vi "Status Update.vi"(8 "error in (no error)":errorcluster, 11 "Stage Controller in":refnum<class "Stage Controller.lvclass">) -> (0 "error out":errorcluster, 3 "Stage Controller out":refnum<class "Stage Controller.lvclass">)   [LabVIEW 2023, in "Stage Controller.lvlib" / "Stage Controller.lvclass"]
uses:
  Stage Controller.lvclass
  Stage Controller.lvclass/Stage Controller.ctl
  <vilib>/ActorFramework/Actor/Actor.lvclass
  Application Messages/Stage Status Msg/Stage Status Msg.lvclass
  Resources/GLOBAL/GLOBAL Experiment Metadata.vi
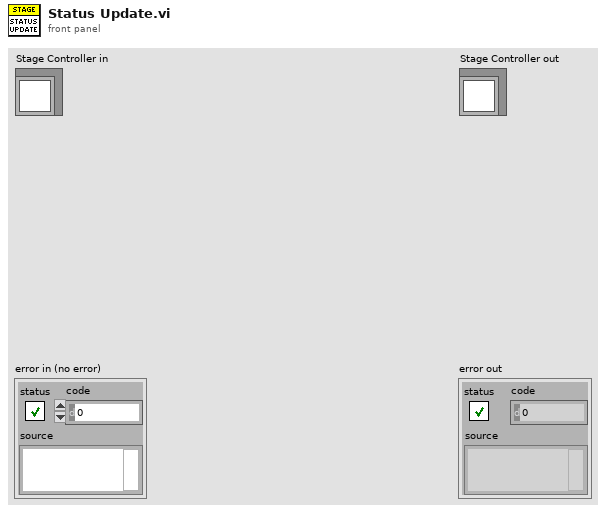
[diagram p1: front panel]
types:
  T1 = cluster{"X (mm)":dbl, "Y (mm)":dbl, "Stage Map":picture}
  T2 = cluster{"Y Min":dbl, "Y Max":dbl, "X Min":dbl, "X Max":dbl}
  T3 = cluster{"top":dbl, "right":dbl, "width":dbl, "height":dbl}
  T4 = typedef "Stage Position.ctl" = cluster{"X (mm)":dbl, "Y (mm)":dbl, "Z (mm)":dbl}
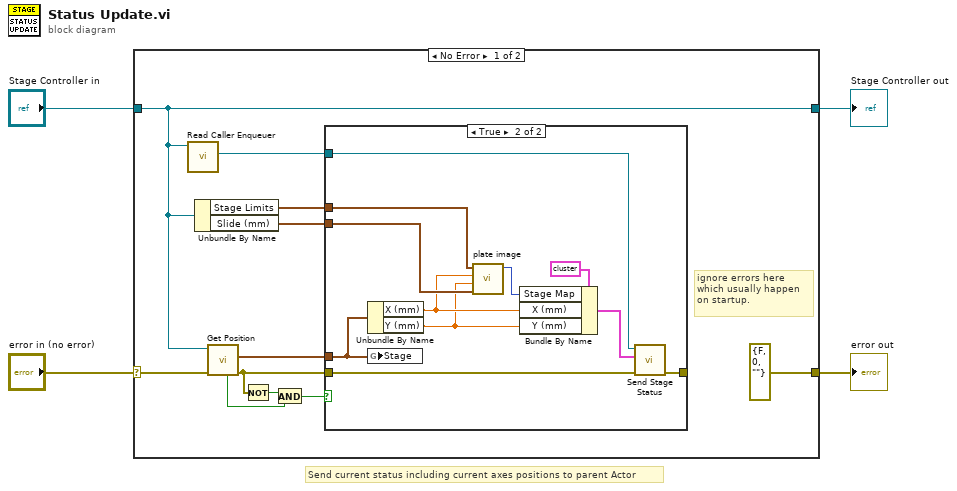
[diagram p0: block diagram]
diagram:
  # "Send current status including current axes positions to parent Actor"
  n1 = case shown="No Error" "error in (no error)" {
    selector: "error in (no error)" -> [w15 w29]
    tunnel: [errorcluster {"status"=FALSE, "code"=0, "source"=""} ("error IO") w29] -> w3
    tunnel: [w9 w28] -> w1
    tunnel: "Stage Controller in" -> [w9 w28]
    frame No Error {
      # "ignore errors here\nwhich usually happen\non startup."
      n2 = call <vilib>:"Read Caller Enqueuer.vi"("Actor"=w9) -> ("Caller Enqueuer"=w14:refnum<class "Message Enqueuer.lvclass">)  [unwired: 10 in]
      n3 = Unbundle By Name(w9) -> ("Stage Limits"=w8:T2, "Slide (mm)"=w5:T3)
      n4 = call-dynamic "Get Position.vi"("error in (no error)"=w15, "Stage Controller in"=w9) -> ("error out"=w13:errorcluster, "Stage Position"=w10:T4, "Value Changed?"=w11:bool)  [unwired: 6 in, 1 out]
      n5 = Not(x=w13) -> (.not. x?=w12:bool)
      n6 = And(x=w12, y=w11) -> (x .and. y?=w7:bool)
      n7 = case shown="True" w7 {
        tunnel: w14 -> [_ w27]
        tunnel: [w16 w25] -> _
        tunnel: w13 -> [w16 w24]
        tunnel: w10 -> [_ w19]
        tunnel: w8 -> [_ w21]
        tunnel: w5 -> [_ w20]
        frame False {
        }
        frame True {
          n8 = Unbundle By Name(w19) -> ("X (mm)"=w18:dbl, "Y (mm)"=w17:dbl)
          n9 = global write "GLOBAL Experiment Metadata.vi" "Stage"(w19) -> ()
          n10 = call "plate image.vi"("Slide (mm)"=w20, "Y (um)"=w17, "X (um)"=w18, "Stage Limits (mm)"=w21) -> ("2D Picture"=w22:picture)  [unwired: 7 in]
          n11 = Bundle By Name(cluster=T1 {"X (mm)"=0.0, "Y (mm)"=0.0, "Stage Map"=bytes[0]} ("Stage Status"), "Stage Map"=w22, "X (mm)"=w18, "Y (mm)"=w17) -> (w26:T1)
          n12 = call "Send Stage Status.vi"("error in (no error)"=w24, "Stage Status"=w26, "Message Enqueuer"=w27) -> ("error out"=w25:errorcluster)  [unwired: 7 in, 1 out]
        }
      }
    }
    frame Error {
    }
  }
  "error out" <- w3
  "Stage Controller out" <- w1
